vi "Elapsed time.vi"(1 "Start time (ms)":u32, 2 "Current time (ms)":u32) -> (0 "Elapsed time":u32)   [LabVIEW 2020]
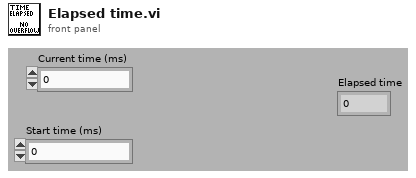
[diagram p1: front panel]
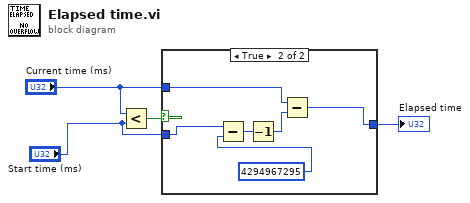
[diagram p0: block diagram]
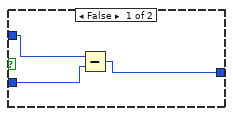
[diagram p2: hidden frame]
diagram:
  n1 = Less?(x="Current time (ms)", y="Start time (ms)") -> (x < y?=w4:bool)
  n2 = case shown="True" w4 {
    tunnel: "Current time (ms)" -> [w7 w13]
    tunnel: "Start time (ms)" -> [w6 w11]
    tunnel: [w5 w12] -> w1
    frame False {
      n3 = Subtract(x=w7, y=w6) -> (x-y=w5:u32)
    }
    frame True {
      n4 = Subtract(x=w11, y=u32 4294967295) -> (x-y=w10:u32)
      n5 = Decrement(x=w10) -> (x-1=w8:u32)
      n6 = Subtract(x=w13, y=w8) -> (x-y=w12:u32)
    }
  }
  "Elapsed time" <- w1
